vi "ConfigureFlowUnit.vi"(0 "object in":refnum<class "CetoniPump.lvclass">, 2 "SyringeSettings":T4={"Prefix"=-3, "TimeUnit"=60, "VolumeUnit"=68} {"VolumeUnit" items=["LITRES"=68]; "TimeUnit" items=["PER_SECOND"=1, "PER_MINUTE"=60, "PER_HOUR"=3600]; "Prefix" items=["UNIT"=0, "DECI"=-1, "CENTI"=-2, "MILLI"=-3, "MICRO"=-6]}, 5 "error in (no error)":errorcluster) -> (14 "object out":refnum<class "CetoniPump.lvclass">, 19 "error out":errorcluster)   [LabVIEW 2024, in "CetoniPump.lvclass"]
uses:
  CetoniPump.lvclass
  Users/Lab user/AppData/Local/CETONI_SDK/lib/labview/labbCAN_Bus_API/SiUnitPrefix.ctl
  Users/Lab user/AppData/Local/CETONI_SDK/lib/labview/labbCAN_Bus_API/TimeUnits.ctl
  Users/Lab user/AppData/Local/CETONI_SDK/lib/labview/labbCAN_Pump_API/VolumeUnits.ctl
  CetoniPump.lvclass/CetoniPump.ctl
  Users/Lab user/AppData/Local/CETONI_SDK/lib/labview/labbCAN_Pump_API/labbCAN_Pump_API.lvlib
  Users/Lab user/AppData/Local/CETONI_SDK/lib/labview/labbCAN_Bus_API/labbCAN_Bus_API.lvlib
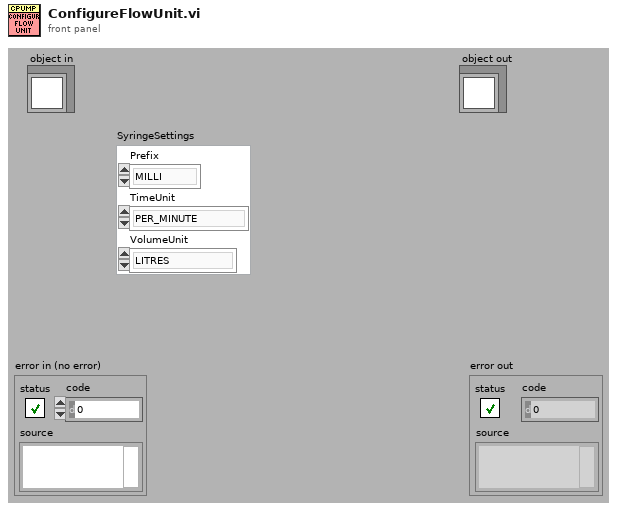
[diagram p1: front panel]
types:
  T1 = typedef "labbCAN_Bus_API.lvlib/SiUnitPrefix.ctl" = i32
  T2 = typedef "labbCAN_Bus_API.lvlib/TimeUnits.ctl" = i32
  T3 = typedef "labbCAN_Pump_API.lvlib/VolumeUnits.ctl" = i32
  T4 = cluster{"Prefix":T1, "TimeUnit":T2, "VolumeUnit":T3}
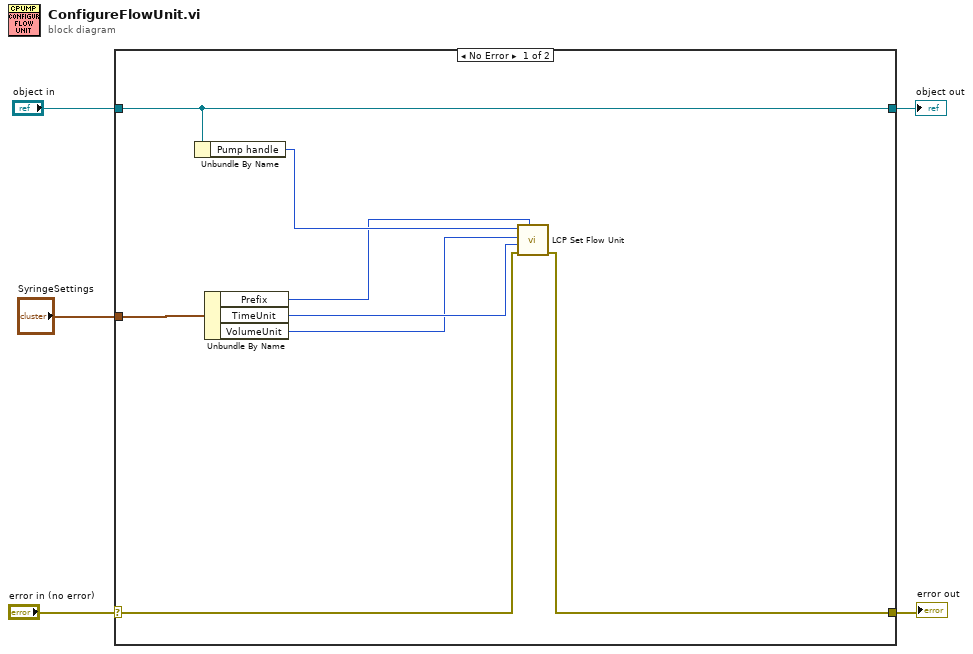
[diagram p0: block diagram]
diagram:
  n1 = case shown="No Error" "error in (no error)" {
    selector: "error in (no error)" -> [w7 w15]
    tunnel: [w6 w15] -> w4
    tunnel: [w13 w14] -> w2
    tunnel: "object in" -> [w13 w14]
    tunnel: "SyringeSettings" -> [w11 _]
    frame No Error {
      n2 = Unbundle By Name(w13) -> ("Pump handle"=w12:i64)
      n3 = Unbundle By Name(w11) -> ("Prefix"=w10:T1, "TimeUnit"=w9:T2, "VolumeUnit"=w8:T3)
      n4 = call "LCP Set Flow Unit.vi"("Prefix"=w10, "error in (no error)"=w7, "TimeUnit"=w9, "VolumeUnit"=w8, "Pump Handle"=w12) -> ("error out"=w6:errorcluster)  [unwired: 6 in]
    }
    frame Error {
    }
  }
  "error out" <- w4
  "object out" <- w2
